vi "RTP_RTSP - EXAMPLE.vi"() -> ()   [LabVIEW 2014]
uses:
  H264 NAL unit.ctl
panel:
  out "SavePath":path
  out "Frame Count":u64
  in  "stop":bool
  out "Duration (sec)":dbl
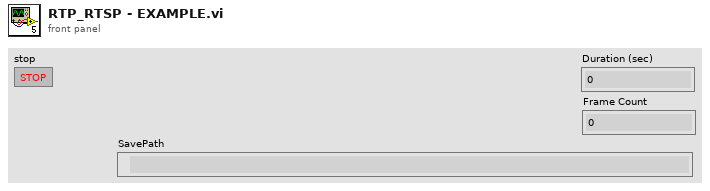
[diagram p1: front panel]
types:
  T1 = typedef "H264 NAL unit.ctl" = cluster{"forbidden_zero_bit":string, "nal_ref_idc":string, "NAL Unit type":string, "Start bit":bool, "End bit":bool, "Data":string}
  T2 = typedef "RTSP Session.ctl" = cluster{"connection ID":refnum<k5>, "Authorization (Basic)":string, "Detailed Stream":string, "DESCRIBE":string, "SETUP":string, "PLAY":string, "TEARDOWN":string}
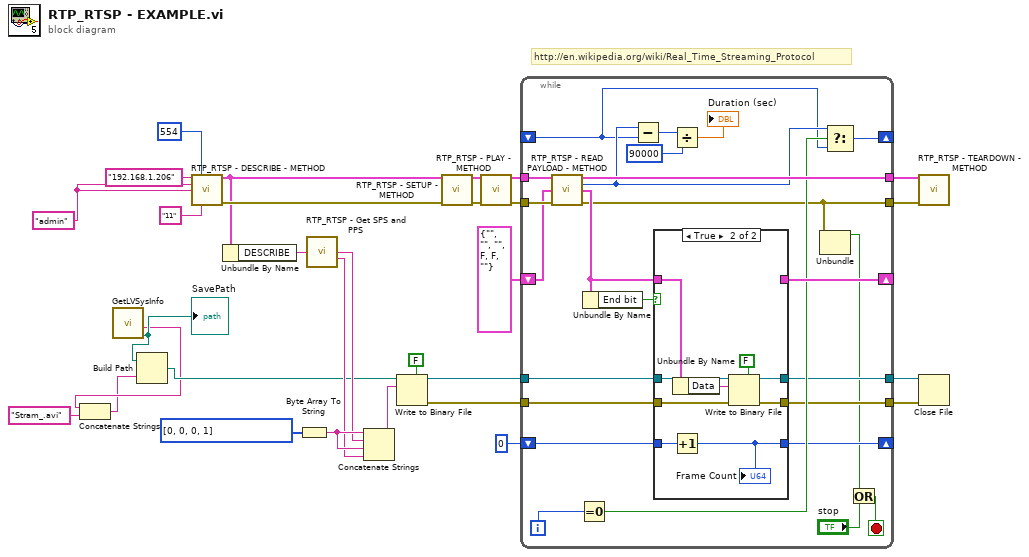
[diagram p0: block diagram]
diagram:
  w8 = "admin" ("uid")
  # "http://en.wikipedia.org/wiki/Real_Time_Streaming_Protocol"
  n1 = call "GetLVSysInfo.vi"() -> ("SavePath"=w5:path, "DateTimeS"=w3:string)  [unwired: 2 in, 8 out]
  "SavePath" <- w5
  n2 = Concatenate Strings(w3, "Stram_.avi" ("string")) -> (w2:string)
  n3 = Build Path(base path=w5, name or relative path=w2) -> (appended path=w4:path)
  n4 = call "RTP_RTSP - DESCRIBE - METHOD.vi"("address"="192.168.1.206", "port"=u16 554, "uid"=w8, "pwd"=w8, "Stream File"="11") -> ("RTSP Session"=w21:T2, "error out"=w30:errorcluster)  [unwired: 9 in]
  n5 = Unbundle By Name(w21) -> ("DESCRIBE"=w20:string)
  n6 = Byte Array To String(unsigned byte array=u8[] [0, 0, 0, 1]) -> (string=w19:string)
  n7 = call "RTP_RTSP - Get SPS and PPS.vi"("DESCRIBE"=w20) -> ("SPS"=w17:string, "PPS"=w16:string)  [unwired: 13 in]
  n8 = Concatenate Strings(w19, w17, w19, w16) -> (w15:string)
  n9 = Write to Binary File(file (use dialog)=w4, data=w15, 5:FALSE ("prepend array or string size? (T)")) -> (refnum out=w13:refnum<file>, error out=w10:errorcluster)  [unwired: 3 in, 1 out]
  n10 = call "RTP_RTSP - SETUP - METHOD.vi"("RTSP Session"=w21, "error in (no error)"=w30) -> ("RTSP Session 2"=w27:T2, "error out"=w28:errorcluster)  [unwired: 12 in]
  n11 = call "RTP_RTSP - PLAY - METHOD.vi"("RTSP Session"=w27, "error in (no error)"=w28) -> ("RTSP Session 2"=w26:T2, "error out"=w25:errorcluster)  [unwired: 12 in]
  n12 = while {
    tunnel: w26 -> [w55]
    tunnel: w25 -> [w54]
    tunnel: [w53] -> w24
    tunnel: [w32] -> w23
    shift-right: [w49] -> _
    shift-left: T1 {"forbidden_zero_bit"="", "nal_ref_idc"="", "NAL Unit type"="", "Start bit"=FALSE, "End bit"=FALSE, "Data"=""} ("H264 NAL unit 2") -> [w52]
    shift-right: [w45] -> _
    shift-left: _ -> [w42]
    tunnel: w13 -> [w41]
    tunnel: [w40] -> w12
    tunnel: [w39] -> w11
    tunnel: w10 -> [w38]
    shift-right: [w35] -> _
    shift-left: u64 0 -> [w36]
    i -> [w46]
    stop <- w33 stop-if-true
    n13 = call "RTP_RTSP - READ PAYLOAD - METHOD.vi"("RTSP Session"=w55, "H264 NAL unit"=w52, "error in (no error)"=w54) -> ("RTSP Session 2"=w53:T2, "timestamp"=w43:u32, "H264 NAL unit 2"=w50:T1, "error out"=w32:errorcluster)  [unwired: 9 in]
    n14 = Equal To 0?(x=w46) -> (x = 0?=w44:bool)
    n15 = Unbundle By Name(w50) -> ("End bit"=w51:bool)
    n16 = Subtract(x=w43, y=w42) -> (x-y=w48:u32)
    n17 = case shown="True" w51 {
      tunnel: w50 -> [w59 w63]
      tunnel: [w59 _] -> w49
      tunnel: w41 -> [w58 w68]
      tunnel: [w58 w67] -> w40
      tunnel: [w57 w65] -> w39
      tunnel: w38 -> [w57 w66]
      tunnel: [w56 w60] -> w35
      tunnel: w36 -> [w56 w61]
      frame False {
      }
      frame True {
        n18 = Increment(x=w61) -> (x+1=w60:u64)
        "Frame Count" <- w60
        n19 = Unbundle By Name(w63) -> ("Data"=w62:string)
        n20 = Write to Binary File(file (use dialog)=w68, data=w62, error in=w66, 5:FALSE ("prepend array or string size? (T)")) -> (refnum out=w67:refnum<file>, error out=w65:errorcluster)  [unwired: 2 in, 1 out]
      }
    }
    n21 = Divide(x=w48, y=u32 90000) -> (x/y=→"Duration (sec)":dbl)
    n22 = Unbundle(w32) -> ("status"=w31:bool)  [unwired: 2 out]
    n23 = Select(t=w43, s=w44, f=w42) -> (s? t:f=w45:u32)
    n24 = Or(x=w31, y="stop") -> (x .or. y?=w33:bool)
  }
  n25 = call "RTP_RTSP - TEARDOWN - METHOD.vi"("RTSP Session"=w24, "error in (no error)"=w23) -> ()  [unwired: 12 in, 2 out]
  n26 = Close File(refnum=w12, error in=w11) -> ()  [unwired: 2 out]
